vi "Msg.vi"(7 "Actor in":refnum<class "LVCAM.lvclass">, 11 "Panel Event Msg in":refnum<class "Panel Event Msg.lvclass">) -> (0 "error out":errorcluster, 1 "Destroy Self?":bool, 5 "Actor out":refnum<class "LVCAM.lvclass">)   [LabVIEW 2021, in "Panel Event.lvlib" / "Panel Event Msg.lvclass"]
uses:
  Panel Event Msg.lvclass
  AAM/AAM/LVCAM/LVCAM.lvclass
  Panel Event/Panel Event.lvclass
  Panel Event Msg.lvclass/Panel Event Msg.ctl
  2de369d9-551b-4d44-a1f9-73fc44f356fa.vi
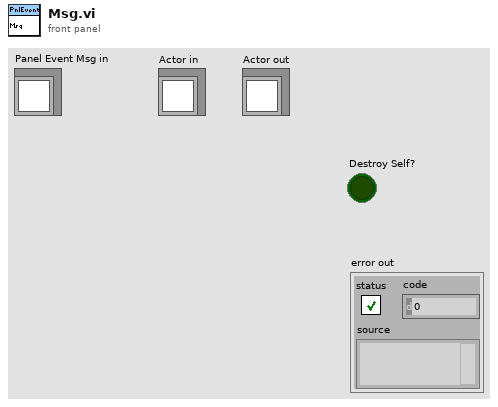
[diagram p1: front panel]
types:
  T1 = typedef "Panel Event.lvlib/Events.ctl" = enum16{"Close Panel", "Show Panel", "Hide Panel"}
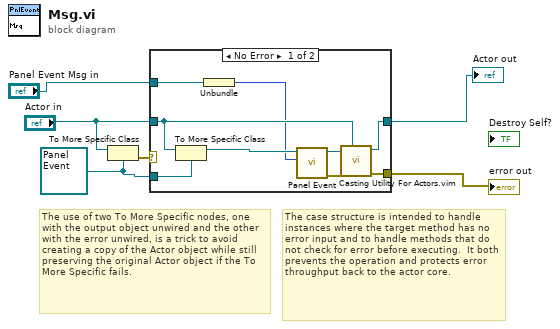
[diagram p0: block diagram]
diagram:
  w1 = refnum<class "Panel Event.lvclass"> refnum ("Panel Event.lvlib:Panel Event.lvclass")
  # "The use of two To More Specific nodes, one with the output object unwired and the other with the error unwired, is a trick to avoid creating a copy of the Actor object while still preserving the original Actor object if the To More Specific fails."
  # "The case structure is intended to handle instances where the target method has no error input and to handle methods that do not check for error before executing.  It both prevents the operation and protects error throughput back to the actor core."
  n1 = To More Specific Class(target class=w1, reference="Actor in") -> (error out=w6:errorcluster)  [unwired: 1 in, 1 out]
  n2 = case shown="No Error" w6 {
    selector: w6 -> [_ w17]
    tunnel: [w12 w17] -> w3
    tunnel: [w13 w16] -> w4
    tunnel: "Actor in" -> [w14 w16]
    tunnel: w1 -> [w15 _]
    tunnel: "Panel Event Msg in" -> [w8 _]
    frame No Error {
      n3 = To More Specific Class(target class=w15, reference=w14) -> (specific class reference=w9:refnum<class "Panel Event.lvclass">)  [unwired: 1 in, 1 out]
      n4 = Unbundle(w8) -> (w7:T1)
      n5 = call-dynamic "Panel Event.vi"("Events"=w7, "Panel Event in"=w9) -> ("error out"=w10:errorcluster, "Panel Event out"=w11:refnum<class "Panel Event.lvclass">)  [unwired: 8 in]
      n6 = call "Casting Utility For Actors.vim"("type"=w14, "error in (no error)"=w10, "Actor in"=w11) -> ("error out"=w12:errorcluster, "Actor out"=w13:refnum<class "LVCAM.lvclass">)  [unwired: 7 in]
    }
    frame Error {
      # "If type check fails, pass the original object out again."
    }
  }
  "error out" <- w3
  "Actor out" <- w4
